vi "3DF-20_Read.vi"() -> ()   [LabVIEW 2022 SP3]
uses:
  <vilib>/Instr/_visa.llb/VISA Configure Serial Port (Instr).vi
panel:
  out "Chart":cluster{"X":dbl, "Y":dbl, "Z":dbl}(graph)
  out "Battery":i32(slide) scale=0.0..3.0
  out "Fz":dbl
  out "Fy":dbl
  out "Fx":dbl
  in  "Serial Port":refnum<visa-resource-name>="COM1"
  out "Response (in HEX)":string
  in  "Stop":bool
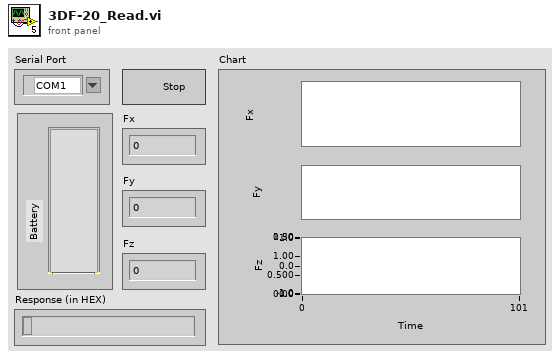
[diagram p1: front panel]
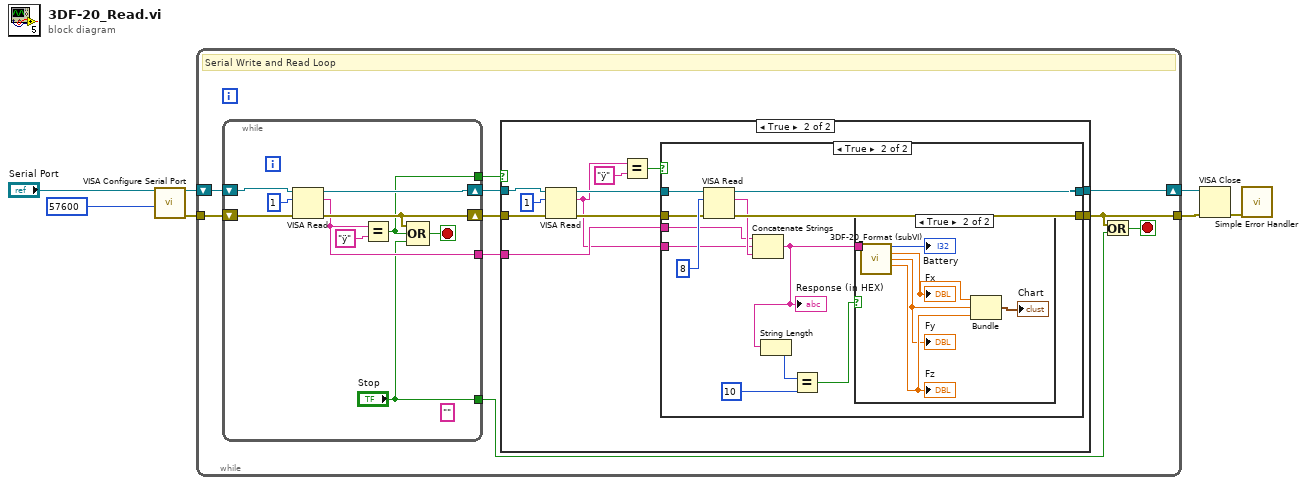
[diagram p0: block diagram]
diagram:
  n1 = call-poly "VISA Configure Serial Port"("VISA resource name"="Serial Port", "baud rate (9600)"=u32 57600) -> ("VISA resource name out"=w2:refnum<visa-resource-name>, "error out"=w3:errorcluster)  [unwired: 8 in, 4 out]
  n2 = while {
    shift-right: [w13] -> w4
    shift-left: w2 -> [w17]
    tunnel: w3 -> [w16]
    tunnel: [w11] -> w5
    stop <- w15 stop-if-true
    # "Serial Write and Read Loop"
    n3 = while {
      shift-right: [w60] -> w14
      shift-left: w17 -> [w59]
      shift-right: [w55] -> w12
      shift-left: w16 -> [w58]
      tunnel: [w53] -> w9
      tunnel: [w52] -> w10
      tunnel: ["Stop"] -> w8
      stop <- w54 stop-if-true
      (unwired) "" ("read buffer")
      n4 = VISA Read(VISA resource name=w59, byte count=u32 1, error in (no error)=w58) -> (VISA resource name out=w60:refnum<visa-resource-name>, read buffer=w52:string, error out=w55:errorcluster)  [unwired: 1 out]
      n5 = Equal?(x=w52, y="ÿ") -> (x = y?=w53:bool)
      n6 = Compound Arithmetic op=OR(w55, w53, "Stop") -> (w54:bool)
    }
    n7 = case shown="True" w9 {
      tunnel: w14 -> [w19 w26]
      tunnel: [w19 w30] -> w13
      tunnel: w12 -> [w18 w25]
      tunnel: [w18 w29] -> w11
      tunnel: w10 -> [_ w28]
      frame False {
      }
      frame True {
        n8 = VISA Read(VISA resource name=w26, byte count=u32 1, error in (no error)=w25) -> (VISA resource name out=w23:refnum<visa-resource-name>, read buffer=w20:string, error out=w24:errorcluster)  [unwired: 1 out]
        n9 = Equal?(x=w20, y="ÿ") -> (x = y?=w21:bool)
        n10 = case shown="True" w21 {
          tunnel: [w32 w44] -> w30
          tunnel: [w31 w43] -> w29
          tunnel: w28 -> [_ w38]
          tunnel: w24 -> [w31 w40]
          tunnel: w23 -> [w32 w39]
          tunnel: w20 -> [_ w37]
          frame False {
          }
          frame True {
            n11 = VISA Read(VISA resource name=w39, byte count=u32 8, error in (no error)=w40) -> (VISA resource name out=w44:refnum<visa-resource-name>, read buffer=w42:string, error out=w43:errorcluster)  [unwired: 1 out]
            n12 = Concatenate Strings(w38, w37, w42) -> (w36:string)
            "Response (in HEX)" <- w36
            n13 = String Length(string=w36) -> (length=w35:i32)
            n14 = Equal?(x=w35, y=10) -> (x = y?=w33:bool)
            n15 = case shown="True" w33 {
              tunnel: w36 -> [_ w50]
              frame False {
              }
              frame True {
                n16 = call "3DF-20_Format (subVI).vi"("raw (hex)"=w50) -> ("BATTERY"=→"Battery":i32, "X"=w46:dbl, "Y"=w47:dbl, "Z"=w48:dbl)  [unwired: 11 in]
                "Fx" <- w46
                "Fy" <- w47
                "Fz" <- w48
                n17 = Bundle("X"=w46, "Y"=w47, "Z"=w48) -> (→"Chart":cluster{"X":dbl, "Y":dbl, "Z":dbl})  [unwired: 1 in]
              }
            }
          }
        }
      }
    }
    n18 = Or(x=w11, y=w8) -> (x .or. y?=w15:bool)
  }
  n19 = VISA Close(VISA resource name=w4, error in (no error)=w5) -> (error out=w6:errorcluster)
  n20 = call <vilib>:"Simple Error Handler.vi"("error in (no error)"=w6) -> ()  [unwired: 1 in, 8 out]
